vi "macro_SimpleMotorFF_Calculate_CalcAccel.vi"   [LabVIEW 2019, in "Trajectory_Library.lvlib"]
uses:
  Trajectory_Library.lvlib
types:
  T1 = typedef "Trajectory_Library.lvlib/SIMPLE_MOTOR_FF.ctl" = cluster{"Ks":dbl, "Kv":dbl, "Ka":dbl, "KnInv":dbl}
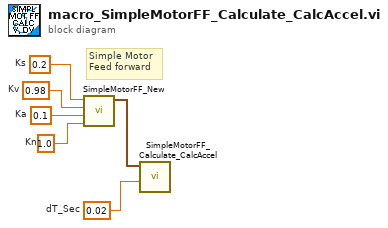
[diagram p0: block diagram]
diagram:
  w1 = 1.0  # Kn
  w2 = 0.02  # dT_Sec
  w4 = 0.2  # Ks
  w5 = 0.98  # Kv
  w6 = 0.1  # Ka
  # "Simple Motor\nFeed forward"
  n1 = call "SimpleMotorFF_New.vi"("Kn"=w1, "Ka"=w6, "Kv"=w5, "Ks"=w4) -> ("SIMPLE_MOTOR_FF"=w3:T1)  [unwired: 7 in]
  n2 = call "SimpleMotorFF_Calculate_CalcAccel.vi"("dT_Sec"=w2, "SIMPLE_MOTOR_FF"=w3) -> ()  [unwired: 9 in, 1 out]
